vi "Set Station Config.vi"(8 "error in (no error)":errorcluster, 10 "Station Config":refnum<class "Station Config.lvclass">, 11 "App Properties in":refnum<class "App Properties.lvclass">) -> (0 "error out":errorcluster, 3 "App Properties out":refnum<class "App Properties.lvclass">)   [LabVIEW 2015, in "Application.lvlib" / "App Properties.lvclass"]
uses:
  App Properties.lvclass
  Station Config/Class/Station Config.lvclass
  App Properties.lvclass/App Properties.ctl
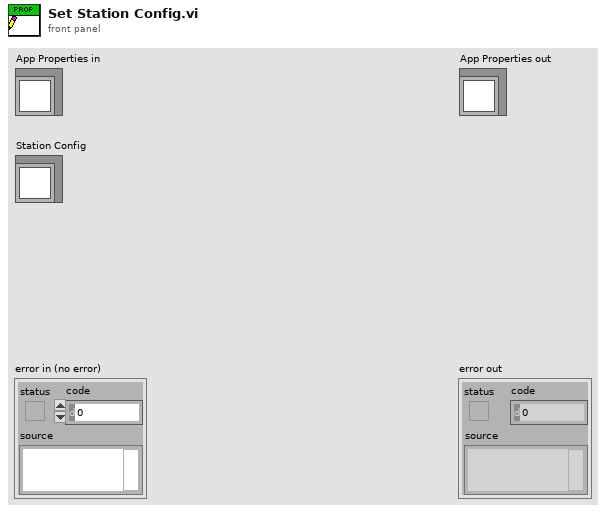
[diagram p1: front panel]
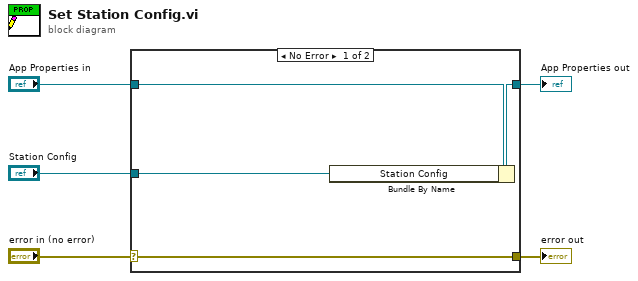
[diagram p0: block diagram]
diagram:
  n1 = case shown="No Error" "error in (no error)" {
    selector: "error in (no error)" -> [w9 w10]
    tunnel: [w9 w10] -> w4
    tunnel: [w7 w11] -> w2
    tunnel: "App Properties in" -> [w8 w11]
    tunnel: "Station Config" -> [w6 _]
    frame No Error {
      n2 = Bundle By Name(cluster=w8, "Station Config"=w6) -> (w7:refnum<class "App Properties.lvclass">)
    }
    frame Error {
    }
  }
  "error out" <- w4
  "App Properties out" <- w2
